vi "Bicycle motor.vi"(7 "Velocity reference":dbl, 8 "Duty cycle in":dbl, 10 "dt":u32, 11 "error in (no error)":errorcluster) -> (0 "Current velocity":dbl, 1 "Accelerate motor":bool, 2 "Duty cycle out":dbl, 3 "error out":errorcluster)   [LabVIEW 2016]
doc: "Inputs\nDuty cycle\ndt\nVelocity reference\n\nOutputs\nCurrent velocity\nAccelerate motor\nDuty cycle out\n\nThis VI controlls the backwheel motor and compares the current velocity with the reference velocity . If the velocity is lower than the reference we increment the duty cycle of the PWM signal, and vice versa if we are above the reference. The dt input is transformed to a velocity in another subVI.\nAccelerate motor indicates if the motor is on or off."
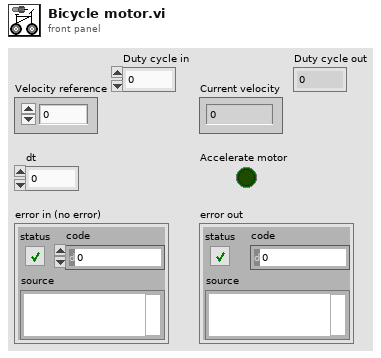
[diagram p1: front panel]
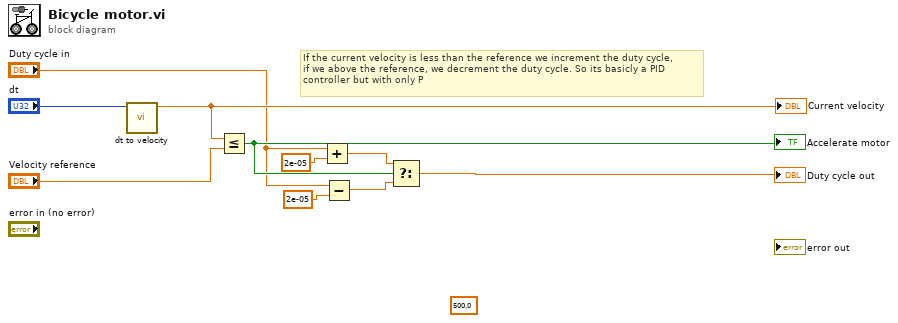
[diagram p0: block diagram]
diagram:
  (unwired) 500.0 ("Frequency [Hz]")
  # "If the current velocity is less than the reference we increment the duty cycle,\nif we above the reference, we decrement the duty cycle. So its basicly a PID\ncontroller but with only P"
  n1 = call "dt to velocity.vi"("dt"="dt") -> ("Velocity (Km/h)"=w4:dbl)  [unwired: 10 in]
  "Current velocity" <- w4
  n2 = Less Or Equal?(x=w4, y="Velocity reference") -> (x <= y?=w8:bool)
  "Accelerate motor" <- w8
  n3 = Add(x="Duty cycle in", y=2e-05) -> (x+y=w5:dbl)
  n4 = Subtract(x="Duty cycle in", y=2e-05) -> (x-y=w3:dbl)
  n5 = Select(t=w5, s=w8, f=w3) -> (s? t:f=→"Duty cycle out":dbl)
